vi "CMD_SETLIGHT.vi"(6 "Gantry in":refnum<class "Gantry.lvclass">, 8 "error in (no error)":errorcluster, 10 "Arguments":string[](array[string]), 11 "gScript Interpreter in":refnum<class "gScript Interpreter.lvclass">) -> (0 "error out":errorcluster, 3 "gScript Interpreter out":refnum<class "gScript Interpreter.lvclass">, 4 "Gantry out":refnum<class "Gantry.lvclass">)   [LabVIEW 2017, in "gScript Interpreter.lvclass"]
uses:
  gScript Interpreter.lvclass
  Shared Components/Gantry Class/Gantry.lvclass
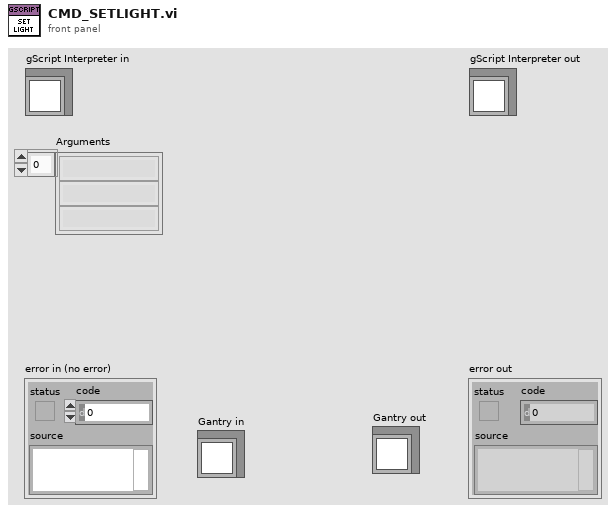
[diagram p1: front panel]
types:
  T1 = typedef "Memory Cell.ctl" = cluster{"type":T2, "x":dbl, "y":dbl, "z":dbl, "w":dbl}
  T2 = typedef "Memory Cell Type Enum.ctl" = enum16{"integer", "float", "vector", "rotation"}
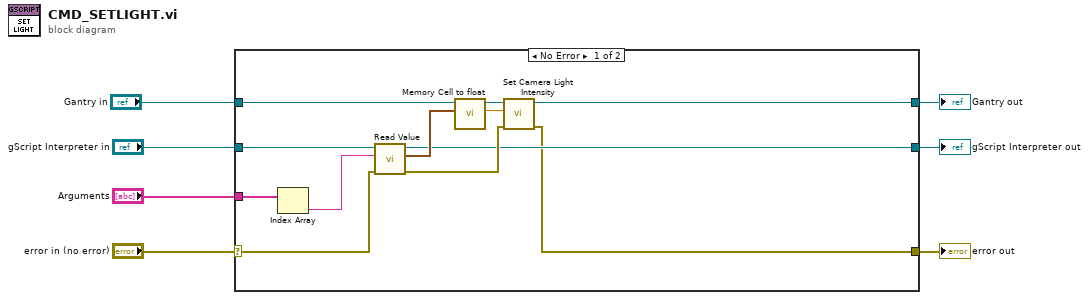
[diagram p0: block diagram]
diagram:
  n1 = case shown="No Error" "error in (no error)" {
    selector: "error in (no error)" -> [w17 w21]
    tunnel: [w8 w21] -> w6
    tunnel: [w9 w20] -> w4
    tunnel: "gScript Interpreter in" -> [w18 w20]
    tunnel: "Arguments" -> [w16 _]
    tunnel: "Gantry in" -> [w13 w19]
    tunnel: [w10 w19] -> w1
    frame No Error {
      n2 = Index Array(array=w16) -> (element=w15:string)  [unwired: 1 in]
      n3 = call-dynamic "Read Value.vi"("error in (no error)"=w17, "String in"=w15, "gScript Interpreter in"=w18) -> ("error out"=w11:errorcluster, "Memory Cell"=w14:T1, "gScript Interpreter out"=w9:refnum<class "gScript Interpreter.lvclass">)  [unwired: 6 in]
      n4 = call "Memory Cell to float.vi"("Memory Cell"=w14) -> ("float out"=w12:dbl)  [unwired: 10 in]
      n5 = call-dynamic "Set Camera Light Intensity.vi"("error in (no error)"=w11, "Intensity"=w12, "Gantry Class in"=w13) -> ("error out"=w8:errorcluster, "Gantry Class out"=w10:refnum<class "Gantry.lvclass">)  [unwired: 7 in]
    }
    frame Error {
    }
  }
  "error out" <- w6
  "gScript Interpreter out" <- w4
  "Gantry out" <- w1
